vi "range.vi"   [LabVIEW 2015]
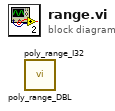
[diagram p0: block diagram]
diagram:
  n1 = call "poly_range_DBL.vi"() -> ()  [unwired: 10 in, 2 out]
  n2 = call "poly_range_I32.vi"() -> ()  [unwired: 10 in, 2 out]
